vi "Ex5-Soling-Eq-using-root.vi"() -> ()   [LabVIEW 2021]
uses:
  <vilib>/httpClient/POSTBuffer.vi
  <vilib>/httpClient/LabVIEWHTTPClient.lvlib
panel:
  out "X2":dbl=-2.0
  out "X1":dbl=3.0
  out "Result":cdb[](array[numeric])=[3.0+0.0i, 2.0-2.4492127076447545e-16i]
  in  "Cluster 2":cluster{"sol_angle":dbl[], "sol_real":dbl[]}={"sol_angle"=[0.0, 3.141592653589793], "sol_real"=[3.0, -2.0]}
  out "body":string="{\"sol_real\":[3.0,-2.0],\"sol_angle\":[0.0,3.141592653589793]}"
  out "headers":string="HTTP/1.1 200 OK\r\ndate: Mon, 02 Mar 2026 11:21:09 GMT\r\nserver: uvicorn\r\ncontent-length: 59\r\ncontent-type: application/json\r\n\r\n"
  in  "Cluster":cluster{"A":dbl, "B":dbl, "C":dbl}={"A"=1.0, "B"=-1.0, "C"=-6.0}
  # "Equation: X^2 - X - 6 = 0"
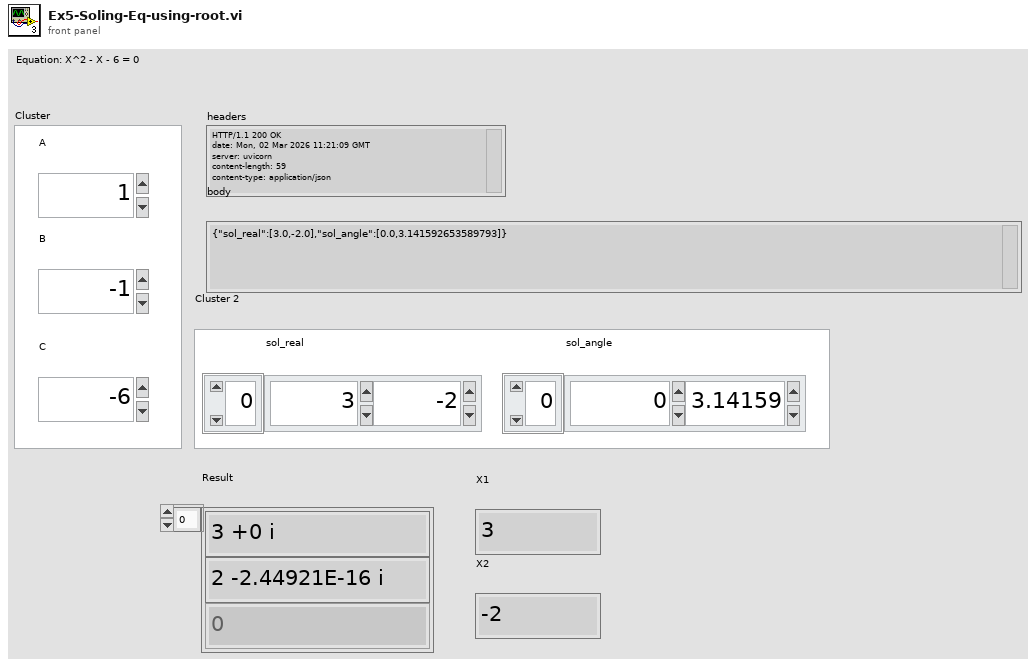
[diagram p1: front panel]
types:
  T1 = typedef "LabVIEWHTTPClient.lvlib/ClientHandle.ctl" = refnum<k1>
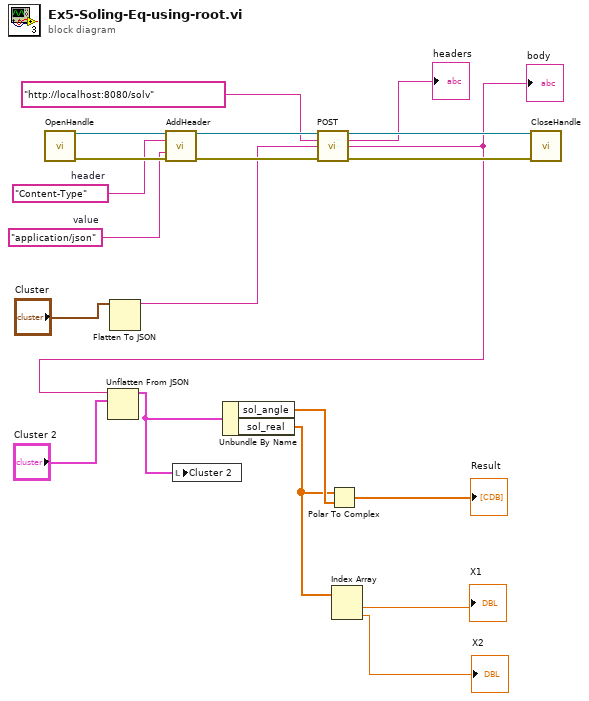
[diagram p0: block diagram]
diagram:
  w13 = "application/json"  # value
  w14 = "Content-Type"  # header
  n1 = call <vilib>:"OpenHandle.vi"() -> ("client handle out"=w20:T1, "error out"=w19:errorcluster)  [unwired: 14 in]
  n2 = Flatten To JSON(anything="Cluster") -> (JSON string=w9:string)  [unwired: 2 in, 1 out]
  n3 = call <vilib>:"AddHeader.vi"("client handle"=w20, "header"=w14, "value"=w13, "error in (no error)"=w19) -> ("client handle out"=w18:T1, "error out"=w17:errorcluster)  [unwired: 10 in]
  n4 = call-poly <vilib>:"POST.vi"("client handle"=w18, "url"="http://localhost:8080/solv", "buffer"=w9, "error in (no error)"=w17) -> ("client handle out"=w16:T1, "headers"=→"headers":string, "body"=w8:string, "error out"=w15:errorcluster)  [unwired: 8 in]
  "body" <- w8
  n5 = Unflatten From JSON(JSON string=w8, type and defaults="Cluster 2") -> (value=w1:cluster{"sol_angle":dbl[], "sol_real":dbl[]})  [unwired: 5 in, 1 out]
  n6 = local write "Cluster 2"(w1) -> ()
  n7 = Unbundle By Name "Unbundle By Name"(w1) -> ("sol_angle"=w6:dbl[], "sol_real"=w4:dbl[])
  n8 = Polar To Complex(1:w6, 2:w4) -> (0:→"Result":cdb[])
  n9 = Index Array "Index Array"(array=w4) -> (element #1=→"X1":dbl, element #2=→"X2":dbl)  [unwired: 2 in]
  n10 = call <vilib>:"CloseHandle.vi"("client handle"=w16, "error in (no error)"=w15) -> ()  [unwired: 13 in, 1 out]
